vi "FGV.vi"(8 "Numeric":i32, 10 "Function":enum16{"Set Value", "Get Value"}(ring), 11 "Value In":string) -> (0 "Numeric 2":i32, 3 "Value out":string)   [LabVIEW 2019, in "Config.lvlib"]
uses:
  Config.lvlib
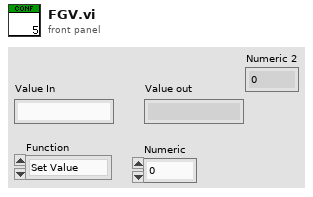
[diagram p1: front panel]
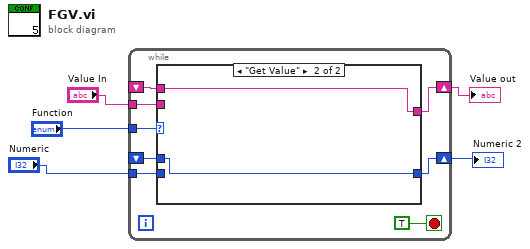
[diagram p0: block diagram]
diagram:
  n1 = while {
    shift-right: [w10] -> w5
    shift-left: _ -> [w9]
    tunnel: "Function" -> [w12]
    tunnel: "Value In" -> [w11]
    tunnel: "Numeric" -> [w8]
    shift-right: [w7] -> w1
    shift-left: _ -> [w6]
    stop <- TRUE stop-if-true
    n2 = case shown="\"Get Value\"" w12 {
      tunnel: w11 -> [w15 _]
      tunnel: [w15 w17] -> w10
      tunnel: w9 -> [_ w17]
      tunnel: w8 -> [w14 _]
      tunnel: [w14 w16] -> w7
      tunnel: w6 -> [_ w16]
      frame "Set Value", Default {
      }
      frame "Get Value" {
      }
    }
  }
  "Value out" <- w5
  "Numeric 2" <- w1
